vi "Example Simple DataBinding.vi"() -> ()   [LabVIEW 2013]
doc: "This examples shows off many of the basic usage patterns of the datagrid."
uses:
  GridColumn/ColumnDefinition.ctl
  GridColumn/ColumnType.ctl
  DataGridView/DataGridView.lvclass
  DataGrid.lvlib
  Events/CellValueChanged/CellValueChanged.lvclass
  Events/CellClick/CellClick.lvclass
  Events/KeyDown/KeyDown.lvclass
  Events/CellDirtyStateChanged/CellDirtyStateChanged.lvclass
  GridColumn/GridColumn.lvclass
  System.Windows.Forms
panel:
  out "cell value":string
  out "Events":string
  in  "# of Rows":i32=15
  in  "ColumnSetup":T1[](array[typedef])=[{"name"="Text", "caption"="Text", "datatype"=enum."string", "Params"="", "AutoSizeMode"=2, "FillWeight"=10.0, "MinWidth"=25, "tooltip"="Text The quick brown fox jumps over the lazy dog"}, {"name"="Details", "caption"="Details", "datatype"=enum."string", "Params"="", "AutoSizeMode"=16, "FillWeight"=100.0, "MinWidth"=150, "tooltip"="Details The quick brown fox jumps over the lazy dog"}, {"name"="Time", "caption"="", "datatype"=enum."timestamp", "Params"="", "AutoSizeMode"=1, "FillWeight"=1.0, "MinWidth"=120, "tooltip"="Time The quick brown fox jumps over the lazy dog"}, {"name"="Selection", "caption"="", "datatype"=enum."combo", "Params"="One|Two|Three", "AutoSizeMode"=6, "FillWeight"=1.0, "MinWidth"=80, "tooltip"="Selection The quick brown fox jumps over the lazy dog"}, {"name"="Function", "caption"="", "datatype"=enum."button", "Params"="", "AutoSizeMode"=6, "FillWeight"=1.0, "MinWidth"=50, "tooltip"="Function The quick brown fox jumps over the lazy dog"}, {"name"="Value", "caption"="", "datatype"=enum."numeric", "Params"="", "AutoSizeMode"=6, "FillWeight"=1.0, "MinWidth"=10, "tooltip"="Value The quick brown fox jumps over the lazy dog"}, {"name"="Active", "caption"="", "datatype"=enum."check", "Params"="", "AutoSizeMode"=6, "FillWeight"=1.0, "MinWidth"=10, "tooltip"=""}, {"name"="Status", "caption"="", "datatype"=enum."image", "Params"="", "AutoSizeMode"=6, "FillWeight"=1.0, "MinWidth"=10, "tooltip"=""}, {"name"="Link", "caption"="", "datatype"=enum."link", "Params"="", "AutoSizeMode"=1, "FillWeight"=100.0, "MinWidth"=50, "tooltip"=""}] {"MinWidth" min=2 step=1; "AutoSizeMode" items=["None"=1, "ColumnHeader"=2, "AllCellsExceptHeader"=4, "AllCells"=6, "DisplayedCellsExceptHeader"=8, "DisplayedCells"=10, "Fill"=16]; "FillWeight" min=1 max=100}
  in  "DataGridView":refnum<k24>(container)
  # "INSTRUCTIONS:\n1. ColumnSetup defines the column types for in the datagrid.\n2. How many rows of generated sample data you want \n3. Run the VI, interactions will show as events"
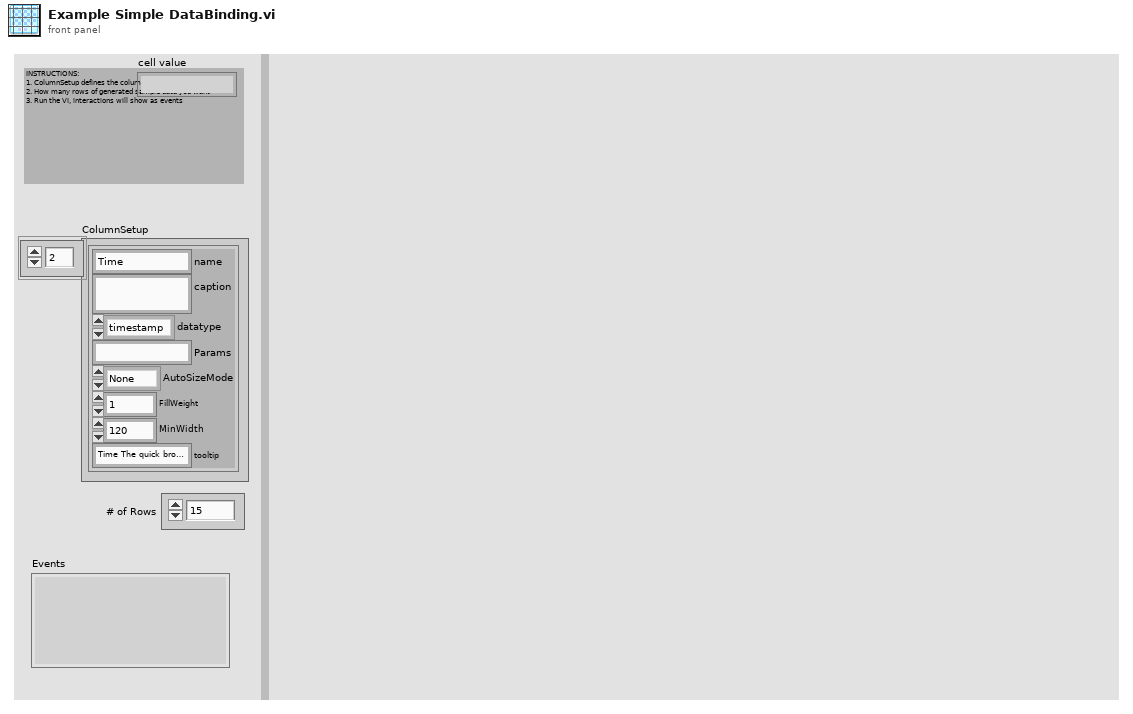
[diagram p1: front panel]
types:
  T1 = typedef "DataGrid.lvlib/GridColumn.lvclass/ColumnDefinition.ctl" = cluster{"name":string, "caption":string, "datatype":T2, "Params":string, "AutoSizeMode":i32, "FillWeight":sgl, "MinWidth":u32, "tooltip":string}
  T2 = typedef "DataGrid.lvlib/GridColumn.lvclass/ColumnType.ctl" = enum16{"string", "image", "check", "numeric", "timestamp", "button", "combo", "link"}
  T3 = cluster{"Alt":bool, "Control":bool, "KeyCode":i32, "KeyData":i32, "KeyValue":i32, "Modifiers":i32, "Shift":bool}
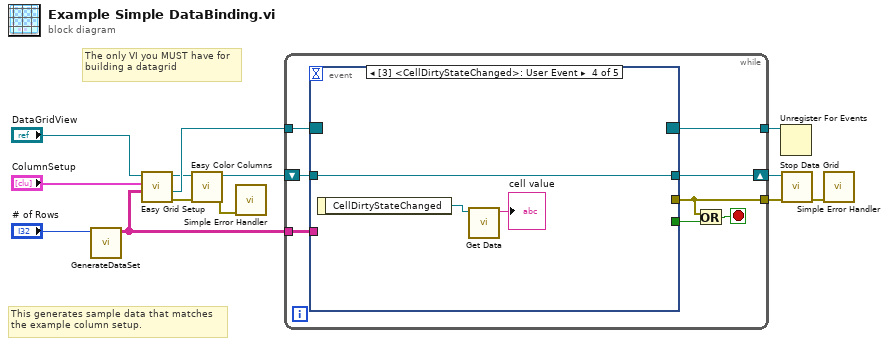
[diagram p0: block diagram]
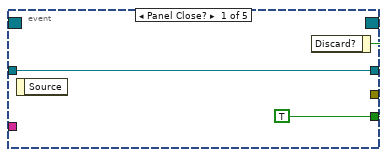
[diagram p2: hidden frame]
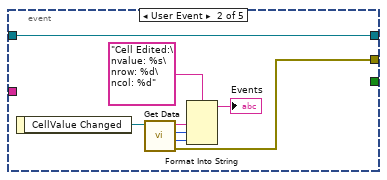
[diagram p3: hidden frame]
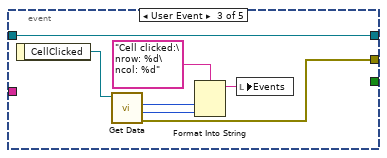
[diagram p4: hidden frame]
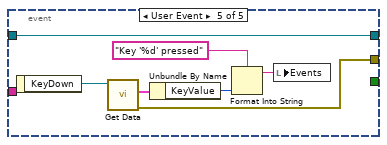
[diagram p5: hidden frame]
diagram:
  # "The only VI you MUST have for building a datagrid"
  # "This generates sample data that matches\nthe example column setup."
  n1 = call "GenerateDataSet.vi"("Records"="# of Rows") -> ("DataGrid"=w3:string[][])  [unwired: 10 in]
  n2 = call "Easy Grid Setup.vi"("DataSource Data"=w3, "ColumnSetup"="ColumnSetup", "DataGridView"="DataGridView") -> ("error out"=w9:errorcluster, "Event Registration Refnum"=w10:refnum<event-registration>, "DataGrid out"=w8:refnum<class "DataGridView.lvclass">)  [unwired: 5 in, 1 out]
  n3 = call "Easy Color Columns.vi"("error in (no error)"=w9, "DataGridView in"=w8) -> ("error out"=w5:errorcluster, "DataGridView out"=w7:refnum<class "DataGridView.lvclass">)  [unwired: 8 in]
  n4 = call <vilib>:"Simple Error Handler.vi"("error in (no error)"=w5) -> ()  [unwired: 4 in, 5 out]
  n5 = while {
    tunnel: w10 -> [w21]
    shift-right: [w19] -> w4
    shift-left: w7 -> [w20]
    tunnel: [w18] -> w6
    tunnel: w3 -> [w17]
    tunnel: [w15] -> w2
    stop <- w14 stop-if-true
    n6 = event shown="[3] <CellDirtyStateChanged>: User Event" {
      selector: w21 -> [_ _ _ _ _]
      dyn-events: [_ _ _ _ _] -> w18
      timeout: _ -> [_ _ _ _ _]
      tunnel: [w23 _ _ _ _] -> w16
      tunnel: w20 -> [w22 w29 w37 w41 w48]
      tunnel: [w22 w29 w37 w41 w48] -> w19
      tunnel: w17 -> [_ _ _ _ _]
      tunnel: [_ w24 w32 _ w42] -> w15
      event Panel Close? {
        w23 = TRUE ("Discard?")
        n7 = event-data() -> ()  [unwired: 1 in, 1 out]
        n8 = event-data("Discard?"=w23) -> ()  [unwired: 1 in, 1 out]
      }
      event User Event {
        n9 = event-data() -> ("CellValue Changed"=w28:refnum<class "Abstract EVENT.lvclass">)  [unwired: 1 in]
        n10 = call "Get Data.vi"("DataGrid.lvlib:Abstract EVENT.lvclass"=w28) -> ("error out"=w24:errorcluster, "column"=w25:i32, "row"=w26:i32, "cell value"=w27:string)  [unwired: 7 in]
        n11 = Format Into String(format string="Cell Edited:\nvalue: %s\nrow: %d\ncol: %d" ("message"), w27, w26, w25) -> (resulting string=→"Events":string)  [unwired: 2 in, 1 out]
      }
      event User Event {
        n12 = event-data() -> ("CellClicked"=w35:refnum<class "Abstract EVENT.lvclass">)  [unwired: 1 in]
        n13 = call "Get Data.vi"("DataGrid.lvlib:Abstract EVENT.lvclass"=w35) -> ("error out"=w32:errorcluster, "column"=w33:i32, "row"=w34:i32)  [unwired: 8 in]
        n14 = Format Into String(format string="Cell clicked:\nrow: %d\ncol: %d" ("message"), w34, w33) -> (resulting string=w38:string)  [unwired: 2 in, 1 out]
        n15 = local write "Events"(w38) -> ()
      }
      event User Event {
        n16 = event-data() -> ("CellDirtyStateChanged"=w40:refnum<class "Abstract EVENT.lvclass">)  [unwired: 1 in]
        n17 = call "Get Data.vi"("DataGrid.lvlib:Abstract EVENT.lvclass"=w40) -> ("cell value"=→"cell value":string)  [unwired: 7 in, 3 out]
      }
      event User Event {
        n18 = event-data() -> ("KeyDown"=w47:refnum<class "Abstract EVENT.lvclass">)  [unwired: 1 in]
        n19 = call "Get Data.vi"("DataGrid.lvlib:Abstract EVENT.lvclass"=w47) -> ("error out"=w42:errorcluster, "output cluster"=w44:T3)  [unwired: 9 in]
        n20 = Unbundle By Name(w44) -> ("KeyValue"=w43:i32)
        n21 = Format Into String(format string="Key '%d' pressed" ("message"), w43) -> (resulting string=w46:string)  [unwired: 2 in, 1 out]
        n22 = local write "Events"(w46) -> ()
      }
    }
    n23 = Or(x=w15, y=w16) -> (x .or. y?=w14:bool)
  }
  n24 = Unregister For Events(event registration refnum=w6) -> ()  [unwired: 1 in, 1 out]
  n25 = call "Stop Data Grid.vi"("error in (no error)"=w2, "DataGridView in"=w4) -> ("error out"=w1:errorcluster)  [unwired: 8 in, 1 out]
  n26 = call <vilib>:"Simple Error Handler.vi"("error in (no error)"=w1) -> ()  [unwired: 4 in, 5 out]
